vi "order_shuffle_stimuli.vi"(10 "Randomize?":bool, 11 "N Stimuli":i32) -> (3 "Riffled":i32[](array[numeric]))   [LabVIEW 2015]
uses:
  <vilib>/Analysis/1siggen.llb/Riffle Array (I32).vi
  <vilib>/Analysis/NI_AALBase.lvlib
panel:
  out "Num Stimuli":i32
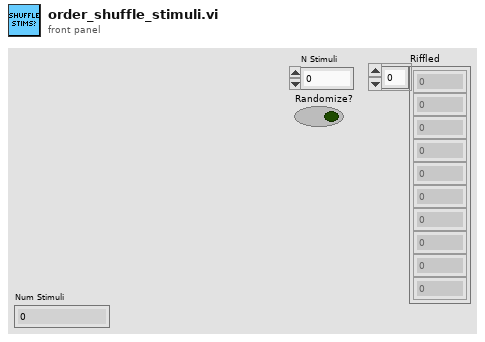
[diagram p1: front panel]
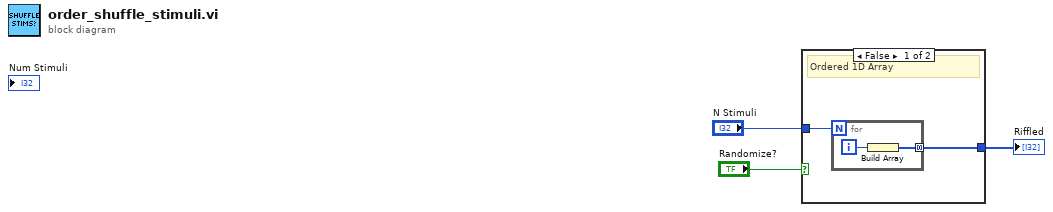
[diagram p0: block diagram]
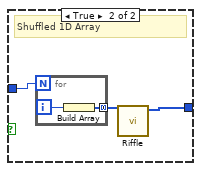
[diagram p2: hidden frame]
diagram:
  n1 = case shown="False" "Randomize?" {
    tunnel: [w5 w9] -> w1
    tunnel: "N Stimuli" -> [w4 w8]
    frame False {
      # "Ordered 1D Array"
      n2 = for {
        N: w4 -> [_]
        tunnel: [w7] -> w5 mode=concatenating
        i -> [w6]
        n3 = Build Array(w6) -> (w7:i32[])
      }
    }
    frame True {
      # "Shuffled 1D Array"
      n4 = for {
        N: w8 -> [_]
        tunnel: [w11] -> w10 mode=concatenating
        i -> [w12]
        n5 = Build Array(w12) -> (w11:i32[])
      }
      n6 = call-poly <vilib>:"Riffle.vi"("X"=w10) -> ("Riffled {X}"=w9:i32[])  [unwired: 8 in, 2 out]
    }
  }
  "Riffled" <- w1
